vi "SCT Handle Attributes Event.vi"(0 "Variable Dialog Controls in":T1, 1 "UsrEvtRef":refnum<user-event>, 3 "attributes":T2, 5 "state variables in":T3, 7 "Event Registration Refnum in":refnum<event-registration>, 11 "error in (no error)":errorcluster, 12 "feature pack info":T8, 14 "main loop broadcast listener":T11) -> (4 "Variable Dialog Controls out":T1, 6 "state variables out":T3, 8 "Event Registration Refnum out":refnum<event-registration>, 10 "done?":bool, 15 "error out":errorcluster)   [LabVIEW 2016]
uses:
  <resource>/dialog/variable/SCT Variable Dialog Controls.ctl
  <resource>/dialog/variable/SCT Broadcast User Event.ctl
  <resource>/dialog/variable/SCT Broadcast.ctl
  <resource>/dialog/variable/SCT Feature Pack Info.ctl
  <resource>/dialog/variable/SCT Message User Event.ctl
  <resource>/dialog/variable/SCT Message.ctl
  <vilib>/variable/Type Descriptor.ctl
  <resource>/dialog/variable/SCT Attributes.ctl
  <resource>/dialog/variable/SCT Attributes Event.ctl
  <resource>/dialog/variable/SCT State Variables.ctl
  <resource>/dialog/variable/SCT Feature State.ctl
  <resource>/dialog/variable/SCT Variable Changes.ctl
  <resource>/dialog/variable/SCT Attribute Changes.ctl
  <vilib>/variable/NI_Variable.lvlib
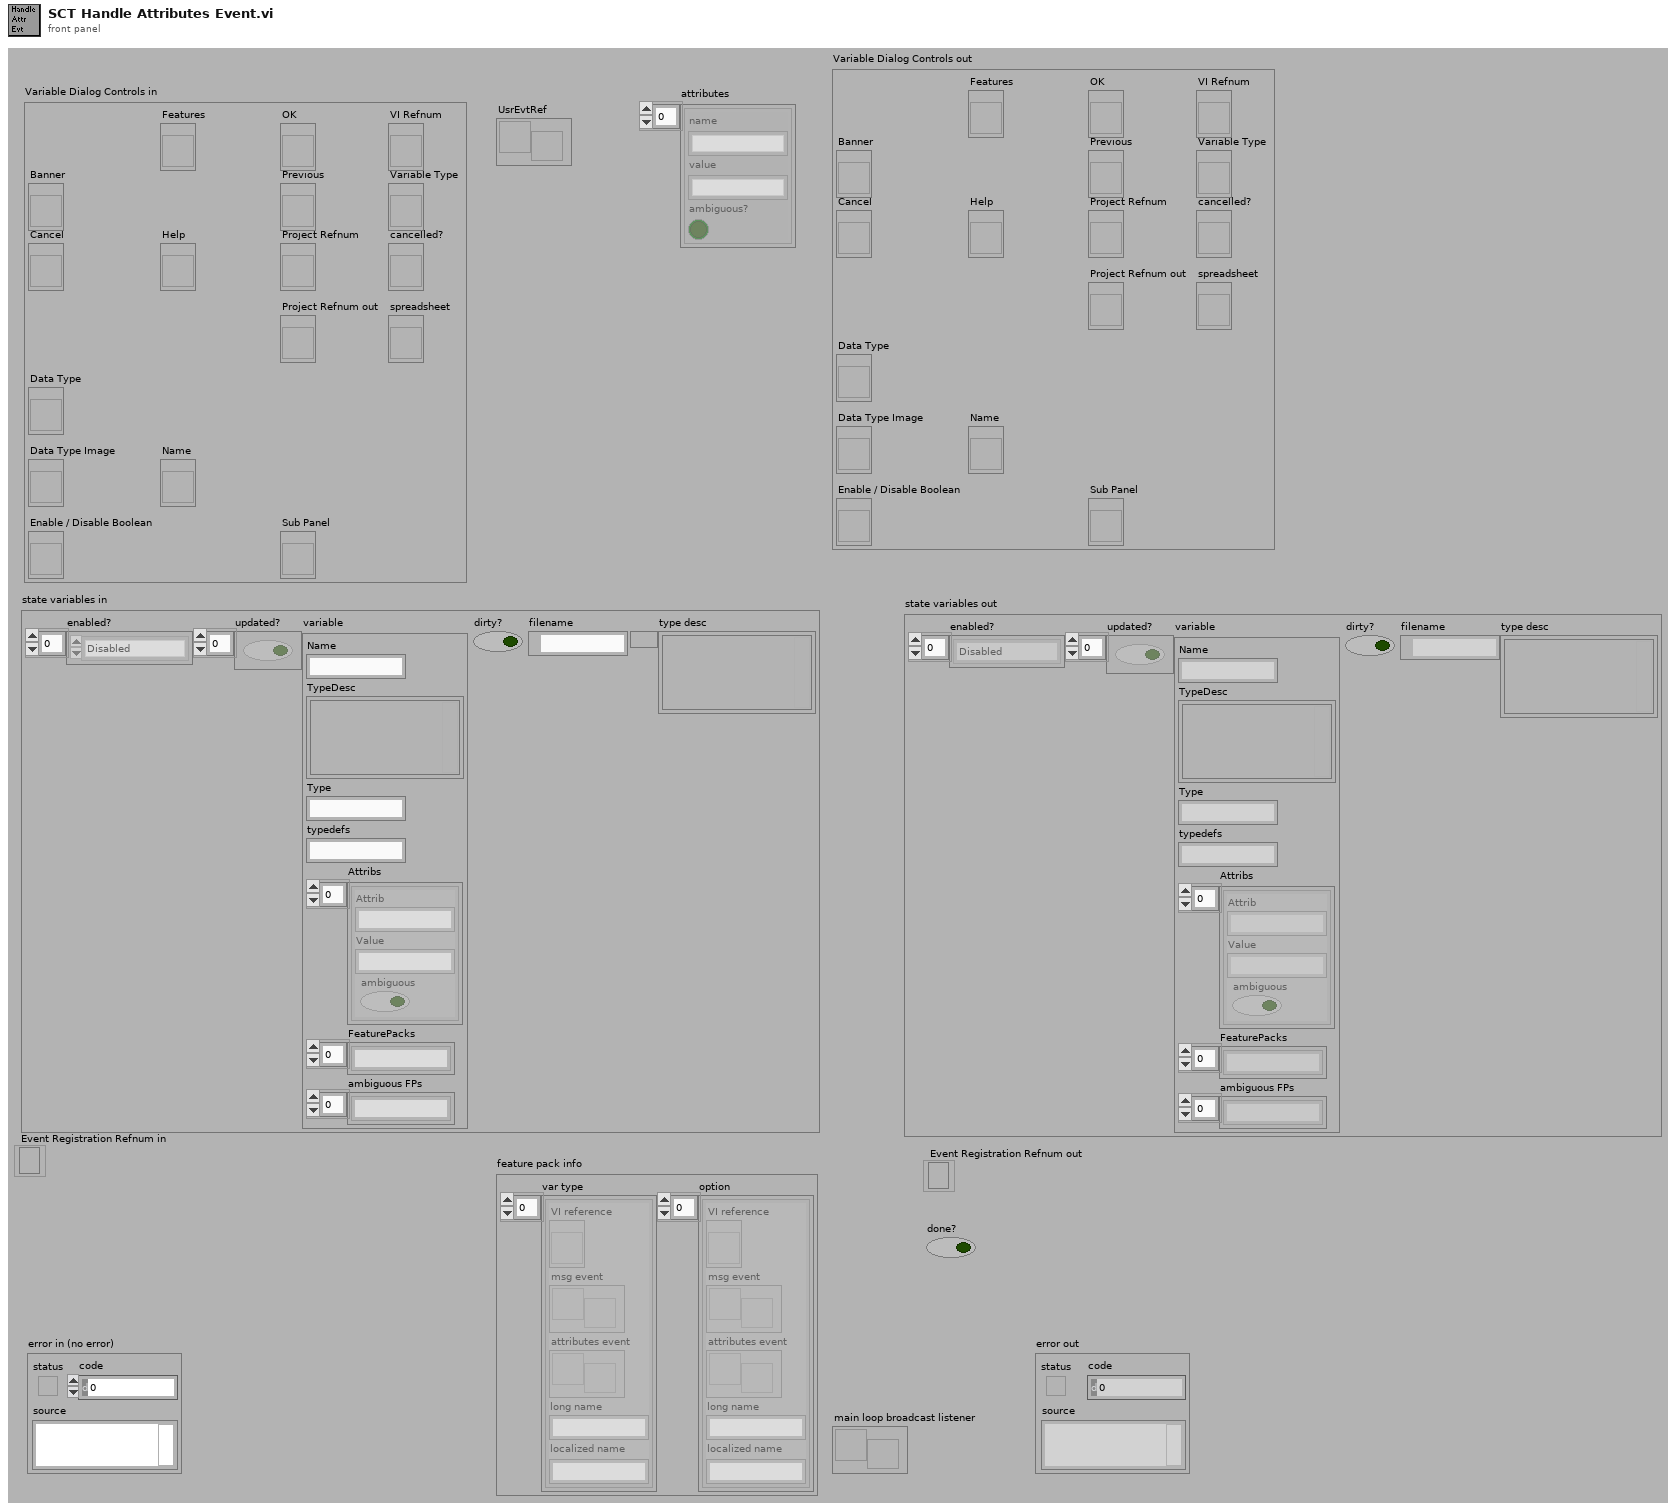
[diagram p1: front panel]
types:
  T1 = typedef "SCT Variable Dialog Controls.ctl" = cluster{"Banner":refnum<vi>, "Cancel":refnum<vi>, "Data Type":refnum<vi>, "Data Type Image":refnum<vi>, "Enable / Disable Boolean":refnum<vi>, "Features":refnum<vi>, "Help":refnum<vi>, "Name":refnum<vi>, "OK":refnum<vi>, "Previous":refnum<vi>, "Project Refnum":refnum<vi>, "Project Refnum out":refnum<vi>, "Sub Panel":refnum<vi>, "VI Refnum":refnum<vi>, "Variable Type":refnum<vi>, "cancelled?":refnum<vi>, "spreadsheet":refnum<vi>}
  T2 = typedef "SCT Attributes.ctl" = cluster{"name":string, "value":string, "ambiguous?":bool}[]
  T3 = typedef "SCT State Variables.ctl" = cluster{"enabled?":T4[], "updated?":bool[], "variable":T5, "dirty?":bool, "filename":path, "type desc":T6}
  T4 = typedef "SCT Feature State.ctl" = enum16{"Disabled", "Enabled", "Ambiguous", "Grayed", "MultiSelectConst"}
  T5 = typedef "SCT Variable Changes.ctl" = cluster{"Name":string, "TypeDesc":T6, "Type":string, "typedefs":string, "Attribs":T7, "FeaturePacks":string[], "ambiguous FPs":string[]}
  T6 = typedef "NI_Variable.lvlib/Type Descriptor.ctl" = cluster{"Variant":variant}
  T7 = typedef "SCT Attribute Changes.ctl" = cluster{"Attrib":string, "Value":string, "ambiguous":bool}[]
  T8 = typedef "SCT Feature Pack Info.ctl" = cluster{"var type":cluster{"VI reference":refnum<vi>, "msg event":T9, "attributes event":T10, "long name":string, "localized name":string}[], "option":cluster{"VI reference":refnum<vi>, "msg event":T9, "attributes event":T10, "long name":string, "localized name":string}[]}
  T9 = typedef "SCT Message User Event.ctl" = refnum<user-event>
  T10 = typedef "SCT Attributes Event.ctl" = refnum<user-event>
  T11 = typedef "SCT Broadcast User Event.ctl" = refnum<user-event>
  T12 = cluster{string, "value":string, "ambiguous?":bool}
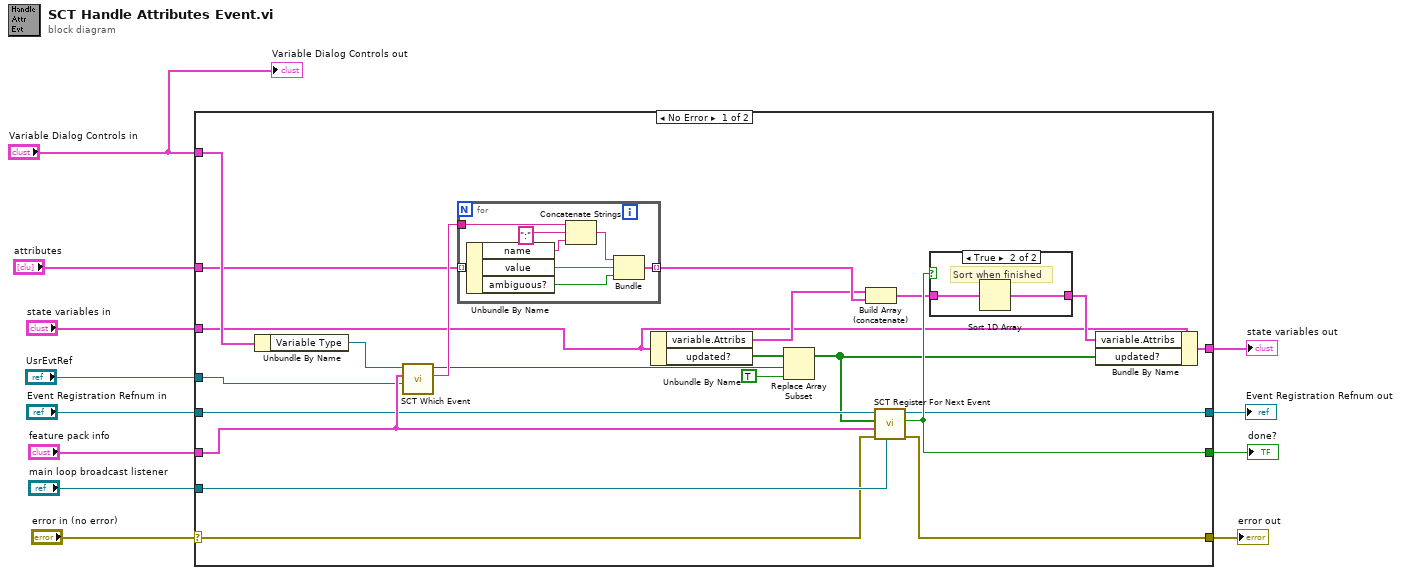
[diagram p0: block diagram]
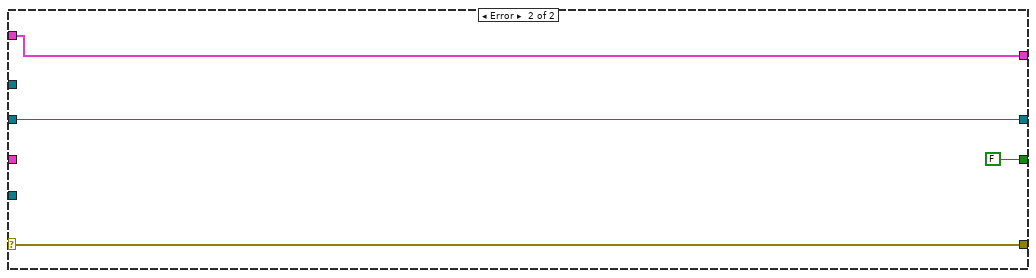
[diagram p3: hidden frame]
diagram:
  n1 = case shown="No Error" "error in (no error)" {
    selector: "error in (no error)" -> [w14 w49]
    tunnel: "Variable Dialog Controls in" -> [w33 _]
    tunnel: [w32 FALSE ("done?")] -> w12
    tunnel: "main loop broadcast listener" -> [w31 _]
    tunnel: "feature pack info" -> [w26 _]
    tunnel: "UsrEvtRef" -> [w25 _]
    tunnel: "Event Registration Refnum in" -> [w24 w47]
    tunnel: [w22 w47] -> w7
    tunnel: [w21 w46] -> w6
    tunnel: "attributes" -> [w16 _]
    tunnel: [w13 w49] -> w3
    tunnel: "state variables in" -> [w15 w46]
    frame No Error {
      n2 = Unbundle By Name(w33) -> ("Variable Type"=w34:refnum<vi>)
      n3 = call <resource>:"SCT Which Event.vi"("UsrEvtRef"=w25, "feature pack info"=w26, "var type ring"=w34) -> ("long name"=w28:string, "updated? index"=w27:i32)  [unwired: 7 in]
      n4 = for {
        tunnel: w16 -> [w45] mode=indexing
        tunnel: w28 -> [w43]
        tunnel: [w39] -> w18 mode=indexing
        n5 = Unbundle By Name(w45) -> ("name"=w44:string, "value"=w40:string, "ambiguous?"=w38:bool)
        n6 = Concatenate Strings(w43, ":", w44) -> (w41:string)
        n7 = Bundle(w41, "value"=w40, "ambiguous?"=w38) -> (w39:T12)  [unwired: 1 in]
      }
      n8 = Unbundle By Name(w15) -> ("variable.Attribs"=w17:T7, "updated?"=w19:bool[])
      n9 = Replace Array Subset(array=w19, new element=TRUE, index=w27) -> (w23:bool[])
      n10 = Build Array (concatenate)(w17, w18) -> (w29:T7)
      n11 = call <resource>:"SCT Register For Next Event.vi"("main loop broadcast listener"=w31, "error in (no error)"=w14, "feature pack info"=w26, "updated?"=w23, "Event Registration Refnum in"=w24) -> ("error out"=w13:errorcluster, "done?"=w32:bool, "Event Registration Refnum out"=w22:refnum<event-registration>)  [unwired: 4 in]
      n12 = case shown="True" w32 {
        tunnel: w29 -> [w35 w37]
        tunnel: [w35 w36] -> w30
        frame False {
        }
        frame True {
          # "Sort when finished"
          n13 = Sort 1D Array(array=w37) -> (sorted array=w36:T7)
        }
      }
      n14 = Bundle By Name(cluster=w15, "variable.Attribs"=w30, "updated?"=w23) -> (w21:T3)
    }
    frame Error {
    }
  }
  "done?" <- w12
  "Event Registration Refnum out" <- w7
  "state variables out" <- w6
  "error out" <- w3
  "Variable Dialog Controls out" <- "Variable Dialog Controls in"
